vi "Agilent SNA Set Power.vi"(4 "Passthrough (T)":bool=TRUE, 6 "Channel":i8=1 min=1 max=99 step=1, 7 "Agilent SNA & SWP":T1, 8 "error in (no error)":errorcluster, 10 "Source Power, dBm (0.0)":dbl, 11 "VISA Resource Names":T2) -> (0 "error out":errorcluster, 3 "dup VISA Resource Names":T2)   [LabVIEW 2011]
doc: "This vi sets the power range. Only works on the HP 8753D."
uses:
  TypeDefs/Agilent SNA VISA.ctl
  TypeDefs/Agilent SNA Instrument Info.ctl
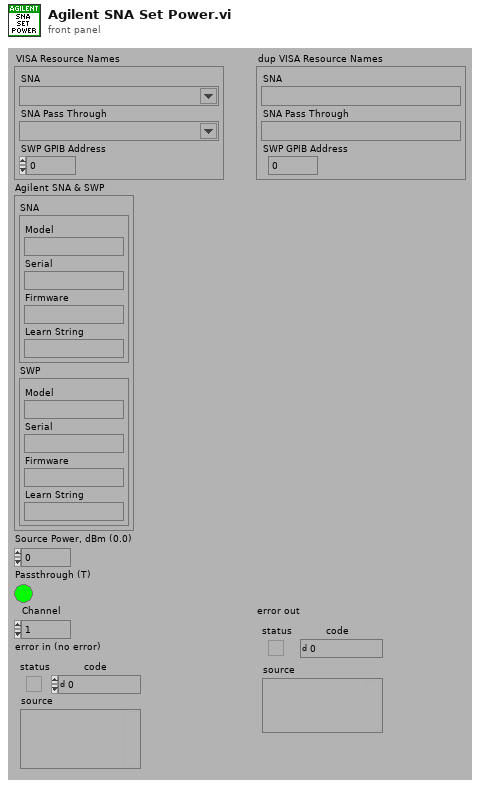
[diagram p1: front panel]
types:
  T1 = typedef "Agilent SNA Instrument Info.ctl" = cluster{"SNA":cluster{"Model":string, "Serial":string, "Firmware":string, "Learn String":string}, "SWP":cluster{"Model":string, "Serial":string, "Firmware":string, "Learn String":string}}
  T2 = typedef "Agilent SNA VISA.ctl" = cluster{"SNA":refnum<visa-resource-name>, "SNA Pass Through":refnum<visa-resource-name>, "SWP GPIB Address":i32}
  T3 = typedef "Agilent SNA Model.ctl" = enum16{"Not Supported", "8757X"}
  T4 = typedef "Agilent SNA SWP Model.ctl" = enum16{"Not Supported", "836XXX", "8375XX", "E82X7D"}
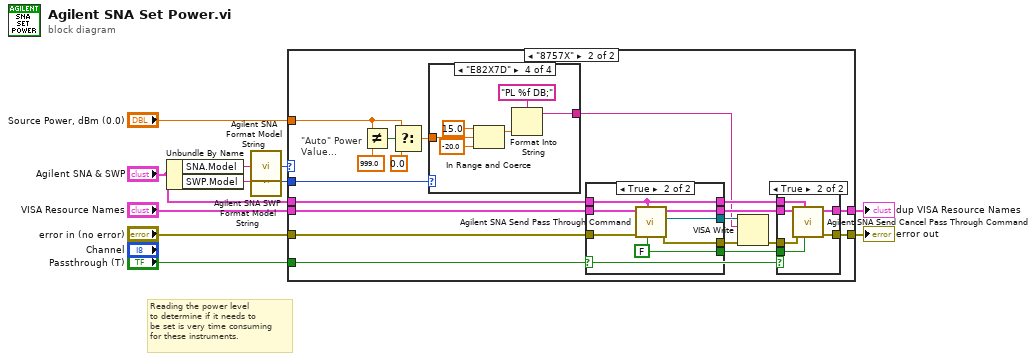
[diagram p0: block diagram]
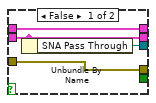
[diagram p4: hidden frame]
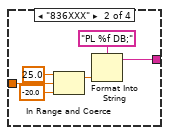
[diagram p6: hidden frame]
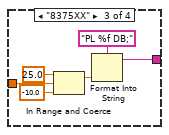
[diagram p7: hidden frame]
diagram:
  # "Reading the power level\nto determine if it needs to\nbe set is very time consuming\nfor these instruments."
  n1 = Unbundle By Name("Agilent SNA & SWP") -> ("SNA.Model"=w8:string, "SWP.Model"=w5:string)
  n2 = call "Agilent SNA Format Model String.vi"("Model String"=w8) -> ("Model"=w9:T3)
  n3 = call "Agilent SNA SWP Format Model String.vi"("Model String"=w5) -> ("Model"=w4:T4)
  n4 = case shown="\"8757X\"" w9 {
    tunnel: [w13 w17] -> w11
    tunnel: "Source Power, dBm (0.0)" -> [_ w29]
    tunnel: "Agilent SNA & SWP" -> [_ w18]
    tunnel: "error in (no error)" -> [w13 w20]
    tunnel: w4 -> [_ w27]
    tunnel: "VISA Resource Names" -> [w12 w19]
    tunnel: [w12 w16] -> w2
    tunnel: "Passthrough (T)" -> [_ w14]
    frame "Not Supported" {
    }
    frame "8757X" {
      # "\"Auto\" Power\nValue..."
      n5 = Not Equal?(x=w29, y=999.0) -> (x != y?=w30:bool)
      n6 = Select(t=w29, s=w30, f=0.0) -> (s? t:f=w28:dbl)
      n7 = case shown="\"E82X7D\"" w27 {
        tunnel: [_ w56 w62 w68] -> w15
        tunnel: w28 -> [_ w54 w60 w66]
        frame "Not Supported" {
        }
        frame "836XXX" {
          n8 = In Range and Coerce(upper limit=25.0, x=w54, lower limit=-20.0) -> (coerced(x)=w55:dbl)  [unwired: 1 out]
          n9 = Format Into String(format string="PL %f DB;", w55) -> (resulting string=w56:string)  [unwired: 2 in, 1 out]
        }
        frame "8375XX" {
          n10 = In Range and Coerce(upper limit=25.0, x=w60, lower limit=-10.0) -> (coerced(x)=w61:dbl)  [unwired: 1 out]
          n11 = Format Into String(format string="PL %f DB;", w61) -> (resulting string=w62:string)  [unwired: 2 in, 1 out]
        }
        frame "E82X7D" {
          n12 = In Range and Coerce(upper limit=15.0, x=w66, lower limit=-20.0) -> (coerced(x)=w67:dbl)  [unwired: 1 out]
          n13 = Format Into String(format string="PL %f DB;", w67) -> (resulting string=w68:string)  [unwired: 2 in, 1 out]
        }
      }
      n14 = case shown="True" w14 {
        tunnel: [w42 w51] -> w22
        tunnel: w20 -> [w43 w50]
        tunnel: w19 -> [w41 w49]
        tunnel: [w43 w48] -> w24
        tunnel: w18 -> [w44 w45]
        tunnel: [w41 w47] -> w25
        tunnel: [_ w46] -> w21
        tunnel: [w44 w45] -> w26
        frame False {
          n15 = Unbundle By Name(w41) -> ("SNA Pass Through"=w42:refnum<visa-resource-name>)
        }
        frame True {
          w46 = FALSE ("SCPI? (F)")
          n16 = call "Agilent SNA Send Pass Through Command.vi"("SCPI? (F)"=w46, "Agilent SNA & SWP"=w45, "error in (no error)"=w50, "VISA Resource Names"=w49) -> ("error out"=w48:errorcluster, "SNA Pass Through"=w51:refnum<visa-resource-name>, "dup VISA Resource Names"=w47:T2)  [unwired: 5 out]
        }
      }
      n17 = VISA Write(VISA resource name=w22, write buffer=w15, error in (no error)=w24) -> (error out=w23:errorcluster)  [unwired: 2 out]
      n18 = case shown="True" w14 {
        tunnel: [w34 w40] -> w17
        tunnel: w25 -> [w33 w39]
        tunnel: w23 -> [w34 w38]
        tunnel: w21 -> [_ w37]
        tunnel: [w33 w36] -> w16
        tunnel: w26 -> [_ w35]
        frame False {
        }
        frame True {
          n19 = call "Agilent SNA Send Cancel Pass Through Command.vi"("SCPI? (F)"=w37, "Agilent SNA & SWP"=w35, "error in (no error)"=w38, "VISA Resource Names"=w39) -> ("error out"=w40:errorcluster, "dup VISA Resource Names"=w36:T2)  [unwired: 6 out]
        }
      }
    }
  }
  "dup VISA Resource Names" <- w2
  "error out" <- w11
